vi "Construct Account.vi"(5 "Account in":refnum<class "Account.lvclass">, 7 "Roles":string[](array[string]), 8 "error in (no error)":errorcluster, 9 "CreatedDate":timestamp, 10 "Active":bool, 11 "Email":string) -> (0 "error out":errorcluster, 3 "Account":refnum<class "Account.lvclass">)   [LabVIEW 2017, in "Account.lvclass"]
uses:
  Account.lvclass
  Account.lvclass/Account.ctl
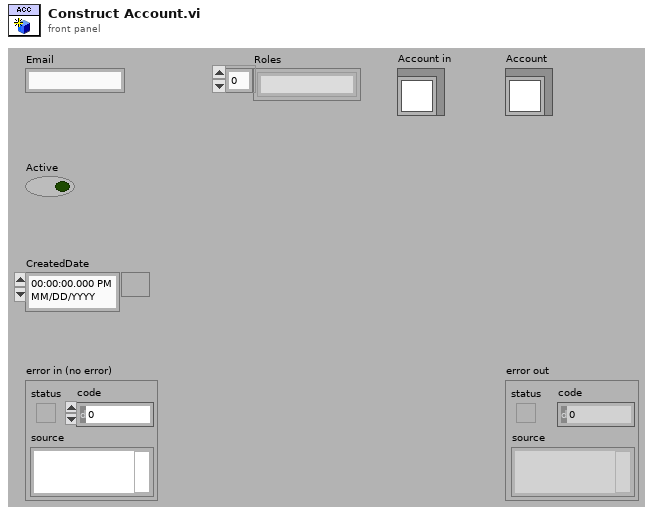
[diagram p1: front panel]
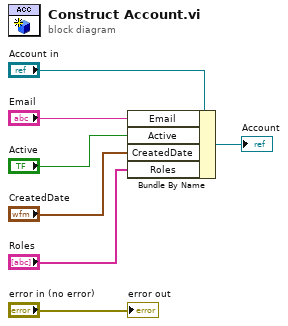
[diagram p0: block diagram]
diagram:
  n1 = Bundle By Name(cluster="Account in", "Email"="Email", "Active"="Active", "CreatedDate"="CreatedDate", "Roles"="Roles") -> (→"Account":refnum<class "Account.lvclass">)
  "error out" <- "error in (no error)"
